vi "Configure Multi Eval Meas List Segment Settings.vi"(0 "VISA resource name":refnum<visa-resource-name>, 1 "Level (0.0)":dbl format="%^.3e", 2 "Band (1)":i32=1, 3 "Evaluation Offset (0)":i32, 5 "Instance (1)":T1=1, 7 "Segment (1)":i32=1, 9 "Segment Length (1)":i32=1, 11 "error in (no error)":errorcluster, 12 "Duplex Mode (FDD)":i32(ring) items=["FDD", "TDD"], 13 "Retrigger Flag (Off)":i32(ring) items=["Off", "On", "IF Power"], 14 "Network Signal (NS01)":i32(ring)=1 items=["NS01"=1, "NS02"=2, "NS03"=3, "NS04"=4, "NS05"=5, "NS06"=6, "NS07"=7, "NS08"=8, "NS09"=9, "NS10"=10, "NS11"=11, "NS12"=12, "NS13"=13, "NS14"=14, "NS15"=15, "NS16"=16, "NS17"=17, "NS18"=18, "NS19"=19, "NS20"=20, "NS21"=21, "NS22"=22, "NS23"=23, "NS24"=24, "NS25"=25, "NS26"=26, "NS27"=27, "NS28"=28, "NS29"=29, "NS30"=30, "NS31"=31, "NS32"=32, "NS35"=35]) -> (4 "VISA resource name out":refnum<visa-resource-name>, 15 "error out":errorcluster)   [LabVIEW 2020, in "Rohde&Schwarz CMWXP NR FR1 Measurement.lvlib"]
doc: "Defines the length and analyzer settings of segment <no>.\n\nAttribute:\nRSCMWXPNRFR1M_ATTR_MULTI_EVAL_MEAS_LIST_SEGMENT_SETTINGS\n\nRemote-control command:\nCONFigure:NRSub:MEAS<i>:LIST:SEGMent<no>:SETup"
uses:
  <instrlib>/Rohde&Schwarz CMWXP NR FR1 Measurement/Rohde&Schwarz CMWXP NR FR1 Measurement.lvlib
  <instrlib>/Rohde&Schwarz CMWXP NR FR1 Measurement/Private/_Instance.ctl
  <instrlib>/Rohde&Schwarz CMWXP NR FR1 Measurement/Private/rsidr_core.llb/rsidr_core.lvlib
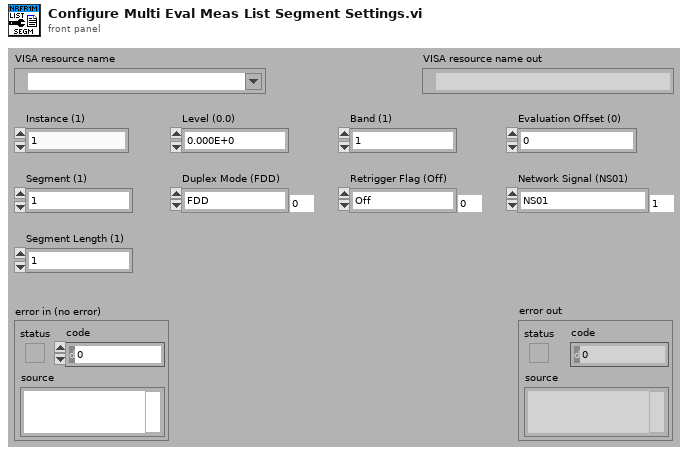
[diagram p1: front panel]
types:
  T1 = typedef "Rohde&Schwarz CMWXP NR FR1 Measurement.lvlib/_Instance.ctl" = i32
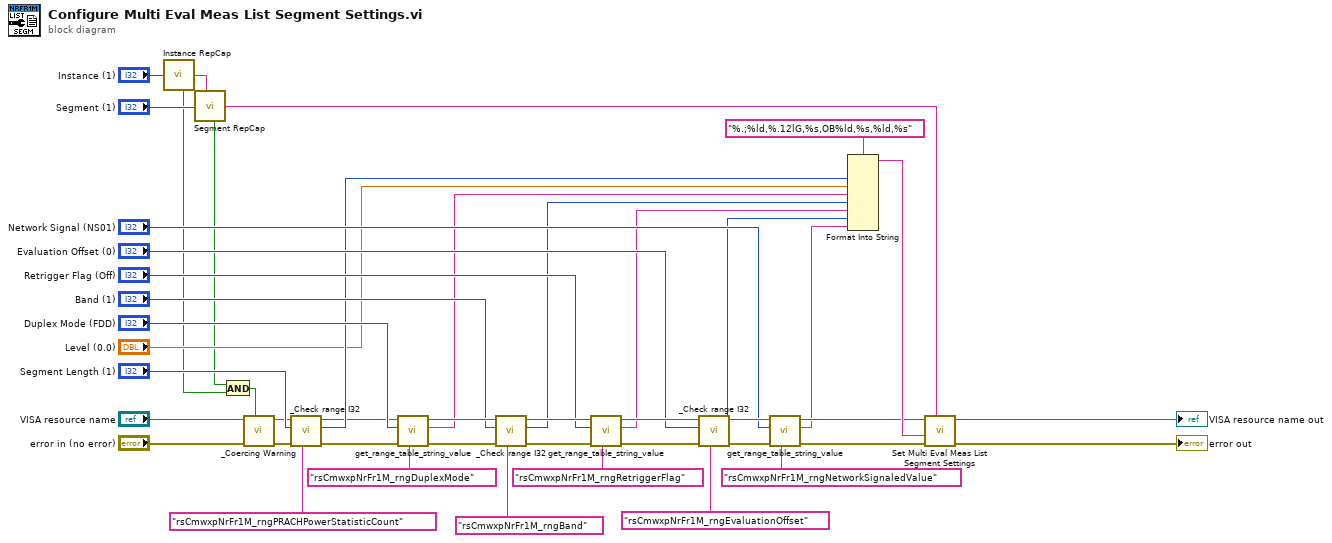
[diagram p0: block diagram]
diagram:
  n1 = call <instrlib>:"Instance RepCap.vi"("Instance In"="Instance (1)") -> ("In Range?"=w2:bool, "RepCap Identifier Out"=w43:string)  [unwired: 1 in]
  n2 = call <instrlib>:"Segment RepCap.vi"("Segment In"="Segment (1)", "RepCap String In (\"\")"=w43) -> ("In Range?"=w1:bool, "RepCap Identifier Out"=w41:string)
  n3 = And(x=w1, y=w2) -> (x .and. y?=w3:bool)
  n4 = call <instrlib>:"_Coercing Warning.vi"("In Range?"=w3, "error in (no error)"="error in (no error)", "VISA resource name"="VISA resource name") -> ("error out"=w5:errorcluster, "VISA resource name out"=w4:refnum<visa-resource-name>)  [unwired: 7 in]
  n5 = call <instrlib>:"_Check range I32.vi"("Range Table Identifier"="rsCmwxpNrFr1M_rngPRACHPowerStatisticCount", "error in (no error)"=w5, "I32 Value In"="Segment Length (1)", "VISA resource name"=w4) -> ("error out"=w13:errorcluster, "I32 Value Out"=w22:i32, "VISA resource name out"=w14:refnum<visa-resource-name>)  [unwired: 5 in]
  n6 = call <instrlib>:"get_range_table_string_value.vi"("Range Table ID in"="rsCmwxpNrFr1M_rngDuplexMode", "error in"=w13, "I32 input"="Duplex Mode (FDD)", "VISA resource name"=w14) -> ("error out"=w39:errorcluster, "String Value out"=w21:string, "VISA resource name out"=w38:refnum<visa-resource-name>)  [unwired: 5 in]
  n7 = call <instrlib>:"_Check range I32.vi"("Range Table Identifier"="rsCmwxpNrFr1M_rngBand", "error in (no error)"=w39, "I32 Value In"="Band (1)", "VISA resource name"=w38) -> ("error out"=w37:errorcluster, "I32 Value Out"=w20:i32, "VISA resource name out"=w36:refnum<visa-resource-name>)  [unwired: 5 in]
  n8 = call <instrlib>:"get_range_table_string_value.vi"("Range Table ID in"="rsCmwxpNrFr1M_rngRetriggerFlag", "error in"=w37, "I32 input"="Retrigger Flag (Off)", "VISA resource name"=w36) -> ("error out"=w35:errorcluster, "String Value out"=w19:string, "VISA resource name out"=w34:refnum<visa-resource-name>)  [unwired: 5 in]
  n9 = call <instrlib>:"_Check range I32.vi"("Range Table Identifier"="rsCmwxpNrFr1M_rngEvaluationOffset", "error in (no error)"=w35, "I32 Value In"="Evaluation Offset (0)", "VISA resource name"=w34) -> ("error out"=w33:errorcluster, "I32 Value Out"=w18:i32, "VISA resource name out"=w32:refnum<visa-resource-name>)  [unwired: 5 in]
  n10 = call <instrlib>:"get_range_table_string_value.vi"("Range Table ID in"="rsCmwxpNrFr1M_rngNetworkSignaledValue", "error in"=w33, "I32 input"="Network Signal (NS01)", "VISA resource name"=w32) -> ("error out"=w29:errorcluster, "String Value out"=w17:string, "VISA resource name out"=w30:refnum<visa-resource-name>)  [unwired: 5 in]
  n11 = Format Into String(format string="%.;%ld,%.12lG,%s,OB%ld,%s,%ld,%s", w22, "Level (0.0)", w21, w20, w19, w18, w17) -> (resulting string=w31:string)  [unwired: 2 in, 1 out]
  n12 = call "Set Multi Eval Meas List Segment Settings"("Repeated Capabilities"=w41, "error in (no error)"=w29, "Multi Eval Meas List Segment Settings ()"=w31, "instrument handle"=w30) -> ("error out"=→"error out":errorcluster, "instrument handle out"=→"VISA resource name out":refnum<visa-resource-name>)  [unwired: 6 in]
